vi "Cargo Intake Immediate with Deadband.vi"(7 "Description":string, 8 "Command Info In":T1, 9 "Deadband Value":dbl=0.01, 11 "Setpoint":dbl) -> (0 "Command Info Out":T1)   [LabVIEW 2018]
doc: "This template includes code for deadband comparision to avoid excessive command scheduling. It is particularly useful for joystick-driven commands.\n\nBe sure to right-click and select New from Template and save with a new command name."
uses:
  <vilib>/Rock Robotics/WPI/Framework/Command Status Info.ctl
  <vilib>/Rock Robotics/WPI/Framework/Completion Status.ctl
  <vilib>/Rock Robotics/WPI/Framework/Completion Notifier.ctl
  Implementation/Cargo Intake Setpoints.ctl
  Implementation/Cargo Intake Operations.ctl
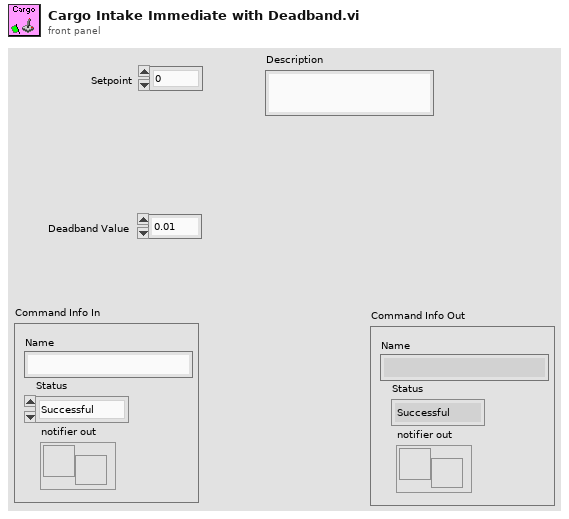
[diagram p1: front panel]
types:
  T1 = typedef "Command Status Info.ctl" = cluster{"Name":string, "Status":T2, "notifier out":T3}
  T2 = typedef "Completion Status.ctl" = enum16{"Successful", "Aborted", "Incomplete"}
  T3 = typedef "Completion Notifier.ctl" = refnum<notifier>
  T4 = typedef "Cargo Intake Setpoints.ctl" = cluster{"Operation":T5, "Setpoint":dbl}
  T5 = typedef "Cargo Intake Operations.ctl" = enum16{"Reserve", "Read Current", "Immediate", "Continuous"}
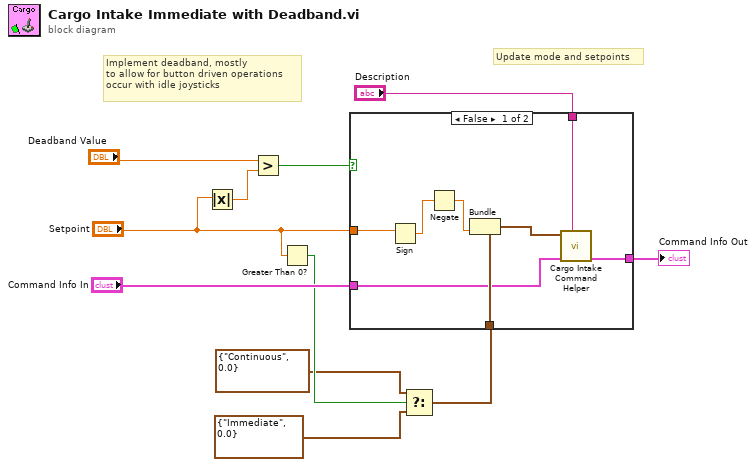
[diagram p0: block diagram]
diagram:
  # "Implement deadband, mostly\nto allow for button driven operations\noccur with idle joysticks"
  # "Update mode and setpoints"
  n1 = Absolute Value(x="Setpoint") -> (abs(x)=w10:dbl)
  n2 = Greater?(x="Deadband Value", y=w10) -> (0:w6:bool)
  n3 = Greater Than 0?(x="Setpoint") -> (x > 0?=w4:bool)
  n4 = Select(t=T4 {"Operation"=enum."Continuous", "Setpoint"=0.0} ("SubSystem Data"), s=w4, f=T4 {"Operation"=enum."Immediate", "Setpoint"=0.0} ("SubSystem Data")) -> (s? t:f=w2:T4)
  n5 = case shown="False" w6 {
    tunnel: "Setpoint" -> [w14 _]
    tunnel: w2 -> [w19 _]
    tunnel: [w18 w20] -> w9
    tunnel: "Command Info In" -> [w17 w20]
    tunnel: "Description" -> [w15 _]
    frame False {
      n6 = Sign(1:w14) -> (0:w13:dbl)
      n7 = Negate(x=w13) -> (-x=w12:dbl)
      n8 = Bundle(cluster=w19, "Setpoint"=w12) -> (w16:T4)  [unwired: 1 in]
      n9 = call "Cargo Intake Command Helper.vi"("Description"=w15, "Command Info In"=w17, "SubSystem Data"=w16) -> ("Command Info Out"=w18:T1)  [unwired: 6 in, 2 out]
    }
    frame True {
    }
  }
  "Command Info Out" <- w9
